vi "Set Shutter.vi"(8 "error in (no error)":errorcluster, 11 "CCDCamera in":refnum<class "iKon-L.lvclass">) -> (0 "error out":errorcluster, 3 "CCDCamera out":refnum<class "iKon-L.lvclass">)   [LabVIEW 2018, in "iKon-L.lvclass"]
doc: "Set the shutter configuration\n\nWith this function, the shutter mode as well as the shutter opening and closing times can be set."
uses:
  iKon-L.lvclass
  C:/Users/Denis/Desktop/S4ACS/S4ACS/Sim_CCD/Sim_CCD.lvclass
  Sim_CCD/Sim_CCD.lvclass
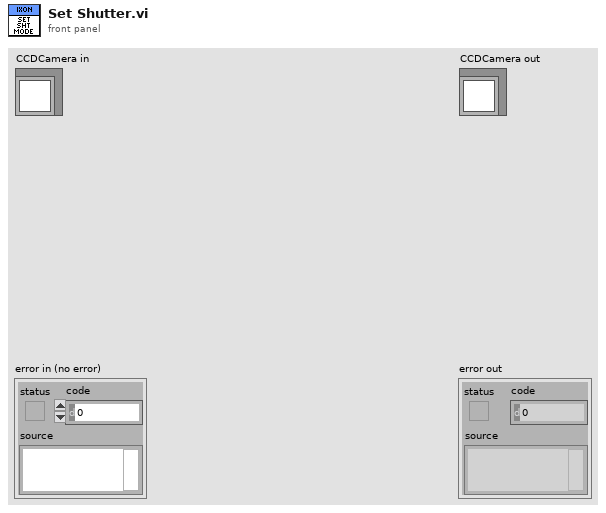
[diagram p1: front panel]
types:
  T1 = cluster{"PREAMP":u16, "READOUT_RATE":u16, "VERTICAL_SHIFT_SPEED":u16, "READ_MODE":u16, "VERTICAL_CLOCK_VOLTAGE":u16, "ACQUISITION_MODE":u16, "AD_CHANNEL":u16, "SHUTTER_TTL":u16, "SHUTTER_OPENING_TIME":u16, "SHUTTER_CLOSING_TIME":u16, "SHUTTER_MODE":u16, "TRIGGER_MODE":u16, "VBIN":u16, "INITIAL_LINE":u16, "INITIAL_COLUMN":u16, "FINAL_LINE":u16, "FINAL_COLUMN":u16, "HBIN":u16}
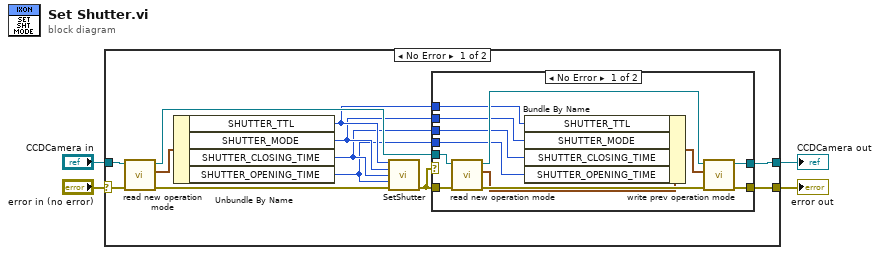
[diagram p0: block diagram]
diagram:
  n1 = case shown="No Error" "error in (no error)" {
    selector: "error in (no error)" -> [w16 w32]
    tunnel: [w11 w32] -> w4
    tunnel: [w12 w31] -> w3
    tunnel: "CCDCamera in" -> [w14 w31]
    frame No Error {
      n2 = call "read new operation mode.vi"("error in (no error)"=w16, "CCDCamera in"=w14) -> ("error out"=w5:errorcluster, "new operation mode"=w15:T1, "CCDCamera out"=w13:refnum<class "iKon-L.lvclass">)  [unwired: 7 in]
      n3 = Unbundle By Name(w15) -> ("SHUTTER_TTL"=w10:u16, "SHUTTER_MODE"=w9:u16, "SHUTTER_CLOSING_TIME"=w8:u16, "SHUTTER_OPENING_TIME"=w7:u16)
      n4 = call <userlib>:"SetShutter.vi"("type"=w10, "mode"=w9, "closingtime"=w8, "openingtime"=w7, "error in (no error)"=w5) -> ("error out"=w6:errorcluster)  [unwired: 9 in, 1 out]
      n5 = case shown="No Error" w6 {
        tunnel: [w27 w30] -> w12
        tunnel: [w25 w29] -> w11
        tunnel: w13 -> [w22 w30]
        tunnel: w6 -> [w21 w29]
        tunnel: w10 -> [w20 _]
        tunnel: w9 -> [w19 _]
        tunnel: w8 -> [w18 _]
        tunnel: w7 -> [w17 _]
        frame No Error {
          n6 = call "read new operation mode.vi"("error in (no error)"=w21, "CCDCamera in"=w22) -> ("error out"=w26:errorcluster, "new operation mode"=w24:T1, "CCDCamera out"=w28:refnum<class "iKon-L.lvclass">)  [unwired: 7 in]
          n7 = Bundle By Name(cluster=w24, "SHUTTER_TTL"=w20, "SHUTTER_MODE"=w19, "SHUTTER_CLOSING_TIME"=w18, "SHUTTER_OPENING_TIME"=w17) -> (w23:T1)
          n8 = call "write prev operation mode.vi"("error in (no error)"=w26, "prev operation mode"=w23, "Simulated_CCD_Camera in"=w28) -> ("error out"=w25:errorcluster, "Simulated_CCD_Camera out"=w27:refnum<class "iKon-L.lvclass">)  [unwired: 7 in]
        }
        frame Error {
        }
      }
    }
    frame Error {
    }
  }
  "error out" <- w4
  "CCDCamera out" <- w3
